vi "ASK 1 bits.vi"() -> ()   [LabVIEW 2010]
panel:
  out "Modulation":dynamicdata(graph)
  out "Démodulation":dynamicdata(graph)
  in  "Tableau":bool[](array[boolean])
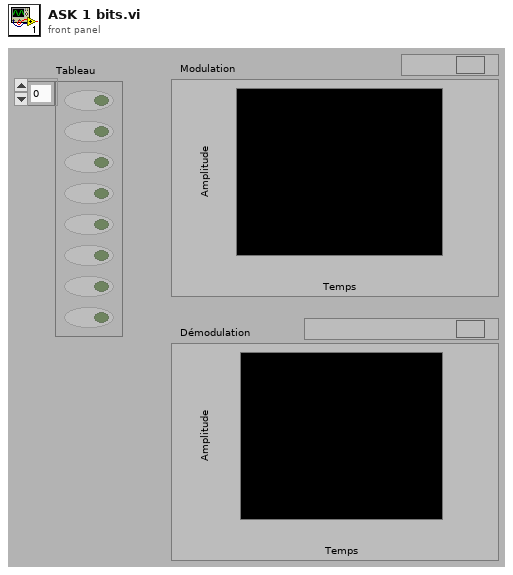
[diagram p1: front panel]
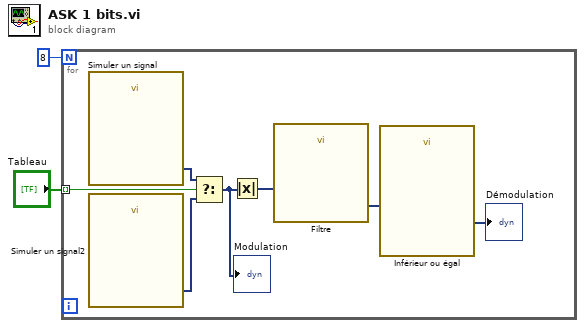
[diagram p0: block diagram]
diagram:
  n1 = for {
    N: 8 -> [_]
    tunnel: "Tableau" -> [w7] mode=indexing
    n2 = call "Simuler un signal"() -> ("Sinus"=w9:dynamicdata)  [unwired: 14 in, 1 out]
    n3 = call "Simuler un signal2"() -> ("Sinus"=w8:dynamicdata)  [unwired: 14 in, 1 out]
    n4 = Select(t=w9, s=w7, f=w8) -> (s? t:f=w3:dynamicdata)
    "Modulation" <- w3
    n5 = Absolute Value(x=w3) -> (abs(x)=w4:dynamicdata)
    n6 = call "Filtre"("Signal"=w4) -> ("Filtered Signal"=w6:dynamicdata)  [unwired: 9 in, 1 out]
    n7 = call "Inférieur ou égal"("Operand 1"=w6) -> ("Result"=→"Démodulation":dynamicdata)  [unwired: 9 in, 1 out]
  }
